vi "AbstractEdge_Create.vi"(0 "reference":refnum<class "AbstractEdge.lvclass">, 5 "error in (no error)":errorcluster) -> (14 "reference out":refnum<class "AbstractEdge.lvclass">, 19 "error out":errorcluster)   [LabVIEW 2016, in "AbstractEdge.lvclass"]
doc: "Creates and initializes a new AbstractEdge object.\n\nThis object should be destroyed using a AbstractEdge destructor VI.\n\n[GOOP 2.1]"
uses:
  <resource>/Framework/Providers/Open_GDS/UML/AbstractEdge_class/AbstractEdge.lvclass
  <resource>/Framework/Providers/Open_GDS/UML/AbstractNode_class/AbstractNode.lvclass
panel:
  # "The input reference should only\nbe wired when this method is called\nby a sub class constructor."
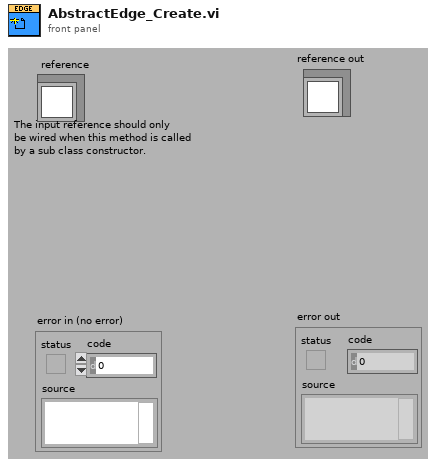
[diagram p1: front panel]
types:
  T1 = typedef "AbstractEdge.lvclass/ObjectAttributes.ctl" = cluster{"start":refnum<class "AbstractNode.lvclass">, "end":refnum<class "AbstractNode.lvclass">}
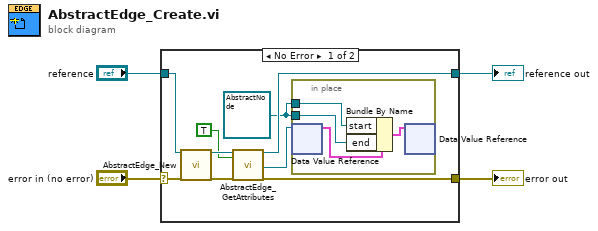
[diagram p0: block diagram]
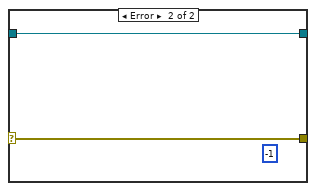
[diagram p2: hidden frame]
diagram:
  n1 = case shown="No Error" "error in (no error)" {
    selector: "error in (no error)" -> [w13 w19]
    tunnel: [w9 w18] -> w4
    tunnel: [w12 w19] -> w3
    tunnel: "reference" -> [w8 w18]
    frame No Error {
      w5 = refnum<class "AbstractNode.lvclass"> refnum ("start")
      n2 = call <resource>:"AbstractEdge_New.vi"("reference in"=w8, "error in (no error)"=w13) -> ("reference out"=w10:refnum<class "AbstractEdge.lvclass">, "error out"=w11:errorcluster)  [unwired: 2 in, 14 out]
      n3 = call <resource>:"AbstractEdge_GetAttributes.vi"("reference in"=w10, "OnlyGetDvrReference(False)"=TRUE, "error in (no error)"=w11) -> ("reference out"=w9:refnum<class "AbstractEdge.lvclass">, "DataRef"=w6:refnum<data-value>, "error out"=w12:errorcluster)  [unwired: 13 in, 1 out]
      n4 = in-place {
        in-place-border: w5 -> [w16]
        in-place-border: w5 -> [w15]
        n5 = in-place-dvr #1(w6) -> (w17:T1)  [unwired: 1 out]
        n6 = Bundle By Name(cluster=w17, "start"=w16, "end"=w15) -> (w14:T1)
        n7 = in-place-dvr #1(w14) -> ()  [unwired: 2 out]
      }
    }
    frame Error {
      (unwired) -1 ("Nr of open handles")
    }
  }
  "error out" <- w3
  "reference out" <- w4
